vi "Write JSON Config.vi"(6 "Pretty Print?":bool, 8 "error in (no error)":errorcluster, 11 "Abs_Type in":refnum<class "Abs_Type.lvclass">) -> (0 "error out":errorcluster, 2 "JSON":string, 3 "Abs_Type out":refnum<class "Abs_Type.lvclass">)   [LabVIEW 2021, in "Abs_Type.lvclass"]
uses:
  Abs_Type.lvclass
  Abs_Type.lvclass/Abs_Type.ctl
  e8f9d266-3841-49b7-afad-ab7c3ba9adfb.vi
  <vilib>/Utility/LVClass/Get LV Class Name.vi
  <vilib>/JDP Science/JSONtext/Variant to JSON Text.vi
  <vilib>/JDP Science/JSONtext/support/Format JSON Object.vi
  <vilib>/JDP Science/JSONtext/LVClass Serializer/JSONtext LVClass Serializer.lvclass
  <vilib>/JDP Science/JSONtext/JSONtext.lvlib
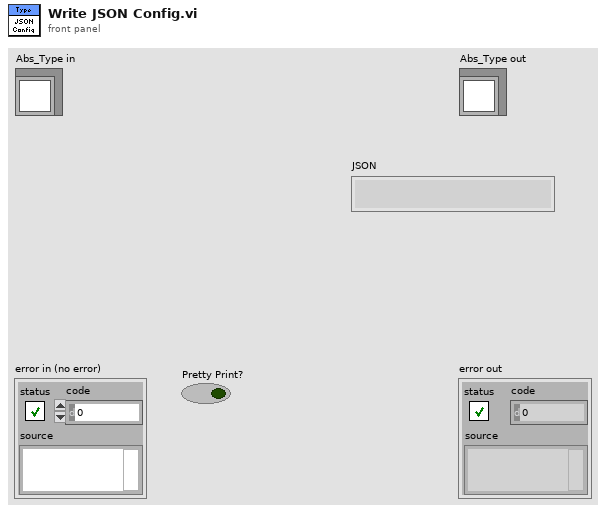
[diagram p1: front panel]
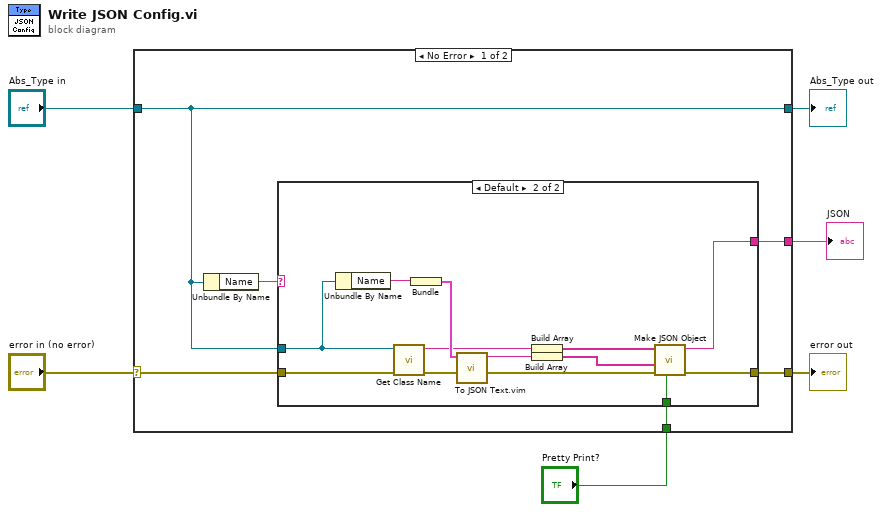
[diagram p0: block diagram]
diagram:
  n1 = case shown="No Error" "error in (no error)" {
    selector: "error in (no error)" -> [w11 w28]
    tunnel: [w12 w28] -> w5
    tunnel: [w8 w27] -> w3
    tunnel: "Abs_Type in" -> [w8 w27]
    tunnel: [w10 _] -> w2
    tunnel: "Pretty Print?" -> [w9 _]
    frame No Error {
      n2 = Unbundle By Name(w8) -> ("Name"=w7:string)
      n3 = case shown="Default" w7 {
        tunnel: [w13 w26] -> w12
        tunnel: w11 -> [w13 w25]
        tunnel: [_ w24] -> w10
        tunnel: w9 -> [_ w23]
        tunnel: w8 -> [_ w15]
        frame "" {
        }
        frame Default {
          n4 = Unbundle By Name(w15) -> ("Name"=w14:string)
          n5 = call "Get Class Name.vi"("error in (no error)"=w25, "Abs_Type in"=w15) -> ("error out"=w21:errorcluster, "class name"=w16:string)  [unwired: 8 in]
          n6 = Bundle("Name"=w14) -> (w22:cluster{"Name":string})  [unwired: 1 in]
          n7 = call "To JSON Text.vim"("error in (no error)"=w21, "Anything"=w22) -> ("error out"=w20:errorcluster, "<JSON>"=w19:string)  [unwired: 8 in]
          n8 = Build Array(w16) -> (w17:string[])
          n9 = Build Array(w19) -> (w18:string[])
          n10 = call <vilib>:"Make JSON Object.vi"("Pretty Print?"=w23, "error in (no error)"=w20, "JSON Items"=w18, "Item Names"=w17) -> ("error out"=w26:errorcluster, "<JSON>"=w24:string)  [unwired: 6 in]
        }
      }
    }
    frame Error {
    }
  }
  "error out" <- w5
  "Abs_Type out" <- w3
  "JSON" <- w2
